vi "Configure Transmit Data.vi"(7 "Virtual Memory Unit in":refnum<class "Virtual Memory Unit.lvclass">, 8 "error in (no error)":errorcluster, 11 "Remote Terminal in":refnum<class "Remote Terminal.lvclass">) -> (0 "error out":errorcluster, 3 "Remote Terminal out":refnum<class "Remote Terminal.lvclass">, 5 "Virtual Memory Unit out":refnum<class "Virtual Memory Unit.lvclass">)   [LabVIEW 2020, in "BCI-1553 API.lvlib" / "Remote Terminal.lvclass"]
doc: "Checks the descriptor table to find the assigned data locations for the transmit data. We then dump all the relevant transmit data to virtual memory."
uses:
  Remote Terminal.lvclass
  Dependencies/Virtual Memory Unit/Virtual Memory Unit.lvclass
  Remote Terminal.lvclass/Remote Terminal.ctl
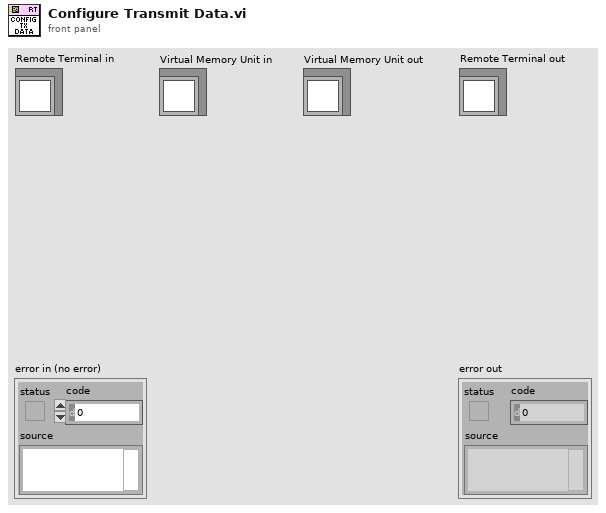
[diagram p1: front panel]
types:
  T1 = typedef "BCI-1553 API.lvlib/Remote Terminal.lvclass/RT CMD Config - Private.ctl" = cluster{"Command Type":T2, "SubAddress":T3, "Word Count\\Mode Code":T4, "Initial Data":u16[], "Data Fields":T5[]}
  T2 = typedef "BCI-1553 API.lvlib/Command Type.ctl" = enum16{"Transmit", "Receive"}
  T3 = typedef "BCI-1553 API.lvlib/Command SubAddress.ctl" = enum16{"Mode Code", "1", "2", "3", "4", "5", "6", "7", "8", "9", "10", "11", "12", "13", "14", "15", "16", "17", "18", "19", "20", "21", "22", "23", "24", "25", "26", "27", "28", "29", "30"}
  T4 = typedef "BCI-1553 API.lvlib/Command Word Count.ctl" = enum16{"1", "2", "3", "4", "5", "6", "7", "8", "9", "10", "11", "12", "13", "14", "15", "16", "17", "18", "19", "20", "21", "22", "23", "24", "25", "26", "27", "28", "29", "30", "31", "32"}
  T5 = typedef "BCI-1553 API.lvlib/Parameter Table Data.ctl" = cluster{"Parameter Name":string, "Base Word":u16, "Address":u16, "Value":u64, "Mask":u16[], "Scaling Info":T6}
  T6 = typedef "BCI-1553 API.lvlib/Scaling Information.ctl" = cluster{"Bit Offset":i32, "Bit Count":i32, "LSB Resolution":dbl, "2's Complement":bool, "Big Endian":bool, "Sign Bit":bool}
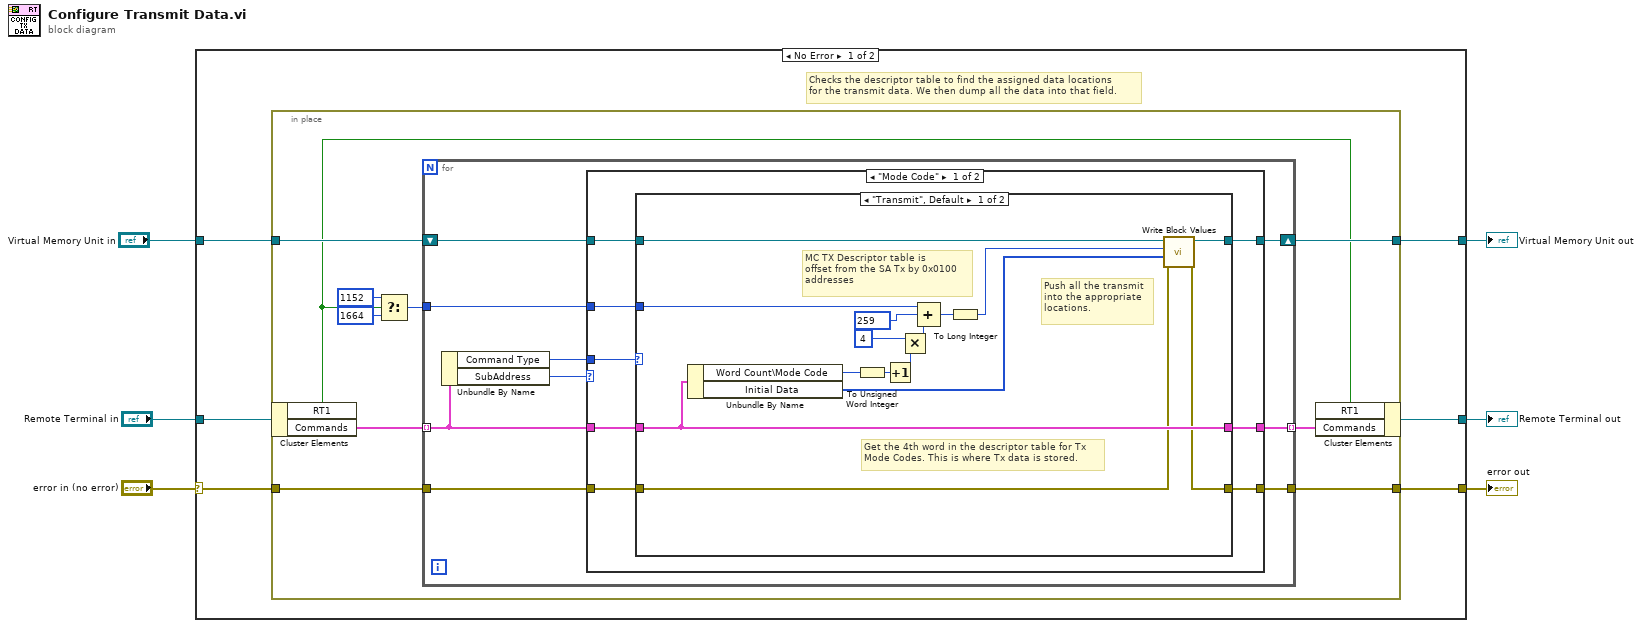
[diagram p0: block diagram]
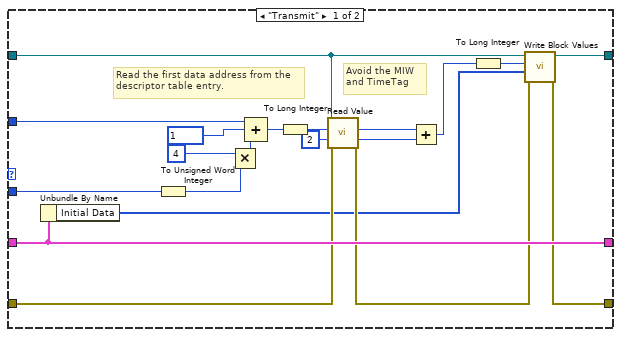
[diagram p4: hidden frame]
diagram:
  n1 = case shown="No Error" "error in (no error)" {
    selector: "error in (no error)" -> [w8 w91]
    tunnel: [w9 w91] -> w5
    tunnel: [w11 w90] -> w3
    tunnel: "Remote Terminal in" -> [w12 w90]
    tunnel: "Virtual Memory Unit in" -> [w10 w89]
    tunnel: [w7 w89] -> w1
    frame No Error {
      # "Checks the descriptor table to find the assigned data locations\nfor the transmit data. We then dump all the data into that field."
      n2 = in-place {
        in-place-border: w10 -> [w16]
        in-place-border: [w19] -> w9
        in-place-border: w8 -> [w18]
        in-place-border: [w15] -> w7
        n3 = in-place-cluster #1(w12) -> ("RT1"=w14:bool, "Commands"=w20:T1[])
        n4 = Select(t=u16 1152 ("Address"), s=w14, f=u16 1664 ("Address")) -> (s? t:f=w17:u16)
        n5 = for {
          tunnel: w20 -> [w26] mode=indexing
          tunnel: [w31] -> w19
          tunnel: w18 -> [w30]
          tunnel: w17 -> [w24]
          shift-right: [w29] -> w15
          shift-left: w16 -> [w28]
          tunnel: [w25] -> w13 mode=indexing
          n6 = Unbundle By Name(w26) -> ("Command Type"=w27:T2, "SubAddress"=w23:T3)
          n7 = case shown="\"Mode Code\"" w23 {
            selector: w23 -> [_ w58]
            tunnel: [w36 w66] -> w31
            tunnel: w30 -> [w35 w65]
            tunnel: [w39 w64] -> w29
            tunnel: w28 -> [w38 w63]
            tunnel: w27 -> [w37 w62]
            tunnel: w26 -> [w33 w61]
            tunnel: [w34 w60] -> w25
            tunnel: w24 -> [w32 w59]
            frame "Mode Code" {
              n8 = case shown="\"Transmit\", Default" w37 {
                tunnel: [w44 w57] -> w39
                tunnel: w38 -> [w45 w57]
                tunnel: [w40 w56] -> w36
                tunnel: w35 -> [w41 w56]
                tunnel: [w42 w55] -> w34
                tunnel: w33 -> [w42 w55]
                tunnel: w32 -> [w43 _]
                frame "Transmit", Default {
                  # "MC TX Descriptor table is\noffset from the SA Tx by 0x0100\naddresses"
                  # "Get the 4th word in the descriptor table for Tx\nMode Codes. This is where Tx data is stored."
                  # "Push all the transmit\ninto the appropriate\nlocations."
                  n9 = Unbundle By Name(w42) -> ("Word Count\\Mode Code"=w51:T4, "Initial Data"=w50:u16[])
                  n10 = To Unsigned Word Integer(number=w51) -> (unsigned 16bit integer=w47:u16)
                  n11 = Increment(x=w47) -> (x+1=w46:u16)
                  n12 = Multiply(x=u16 4 ("y"), y=w46) -> (x*y=w52:u16)
                  n13 = Compound Arithmetic op=ADD(w43, u16 259 ("Address"), w52) -> (w48:u16)
                  n14 = To Long Integer(number=w48) -> (32bit integer=w49:i32)
                  n15 = call "Write Block Values.vi"("error in (no error)"=w41, "Write Block"=w50, "Start Index"=w49, "Virtual Memory Unit in"=w45) -> ("error out"=w40:errorcluster, "Virtual Memory Unit out"=w44:refnum<class "Virtual Memory Unit.lvclass">)  [unwired: 6 in]
                }
                frame "Receive" {
                }
              }
            }
            frame Default {
              n16 = case shown="Default" w62 {
                tunnel: [w74 w88] -> w66
                tunnel: w65 -> [w76 w88]
                tunnel: [w77 w87] -> w64
                tunnel: w63 -> [w78 w87]
                tunnel: w61 -> [w82 w86]
                tunnel: [w82 w86] -> w60
                tunnel: w59 -> [w81 _]
                tunnel: w58 -> [w68 _]
                frame "Transmit" {
                  # "Avoid the MIW\nand TimeTag"
                  # "Read the first data address from the\ndescriptor table entry."
                  n17 = Unbundle By Name(w82) -> ("Initial Data"=w72:u16[])
                  n18 = To Unsigned Word Integer(number=w68) -> (unsigned 16bit integer=w67:u16)
                  n19 = Multiply(x=u16 4 ("y"), y=w67) -> (x*y=w83:u16)
                  n20 = Compound Arithmetic op=ADD(w81, u16 1 ("Address"), w83) -> (w80:u16)
                  n21 = To Long Integer(number=w80) -> (32bit integer=w79:i32)
                  n22 = call "Read Value.vi"("error in (no error)"=w76, "Index"=w79, "Virtual Memory Unit in"=w78) -> ("error out"=w75:errorcluster, "Value"=w70:u16)  [unwired: 7 in]
                  n23 = Add(x=w70, y=u16 2) -> (x+y=w69:u16)
                  n24 = To Long Integer(number=w69) -> (32bit integer=w73:i32)
                  n25 = call "Write Block Values.vi"("error in (no error)"=w75, "Write Block"=w72, "Start Index"=w73, "Virtual Memory Unit in"=w78) -> ("error out"=w74:errorcluster, "Virtual Memory Unit out"=w77:refnum<class "Virtual Memory Unit.lvclass">)  [unwired: 6 in]
                }
                frame Default {
                  # "When it's not a transmit subaddress command\nor a mode code transmit, do nothing."
                }
              }
            }
          }
        }
        n26 = in-place-cluster #1("RT1"=w14, "Commands"=w13) -> (w11:refnum<class "Remote Terminal.lvclass">)
      }
    }
    frame Error {
    }
  }
  "error out" <- w5
  "Remote Terminal out" <- w3
  "Virtual Memory Unit out" <- w1
